vi "LV String to MRC String.vi"(11 "LV String":string) -> (3 "MRC String":T1)   [LabVIEW 2026, in "MrcLib.lvlib"]
uses:
  MrcLib.lvlib
  FRC_NetworkTablesLV.so
  Types/MRC String.ctl
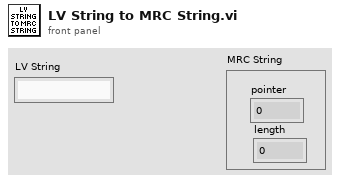
[diagram p1: front panel]
types:
  T1 = typedef "MRC String.ctl" = cluster{"pointer":u64, "length":u64}
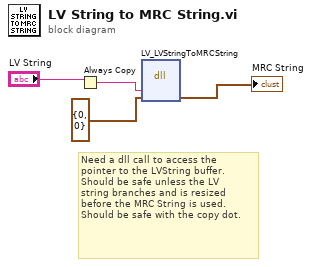
[diagram p0: block diagram]
diagram:
  # "Need a dll call to access the\npointer to the LVString buffer.\nShould be safe unless the LV\nstring branches and is resized\nbefore the MRC String is used.\nShould be safe with the copy dot."
  n1 = Always Copy(1:"LV String") -> (0:w3:string)
  n2 = dll-call lib="FRC_NetworkTablesLV.*" fn="LV_LVStringToMRCString"("lvstr"=w3, "MRC String"=T1 {"pointer"=0, "length"=0}) -> ("MRC String"=→"MRC String":T1)  [unwired: 5 in, 2 out]
